vi "SerialTranscieve.vi"(8 "error in (no error)":errorcluster, 9 "TimeOut(ms)":u32=1000, 10 "ByteArrayToSend":u8[](array[numeric])=[126, 0, 0, 2, 0, 3, 250, 126] format="%x", 11 "VISA resource name":refnum<visa-resource-name>="COM7") -> (0 "error out":errorcluster={"status"=TRUE, "code"=-5000, "source"="Serial Transcieve Timout"}, 1 "return count":u32, 2 "ByteArrayRecieved":u8[](array[numeric]), 3 "VISA resource name out":refnum<visa-resource-name>="COM7")   [LabVIEW 2019]
panel:
  out "Numeric":i32
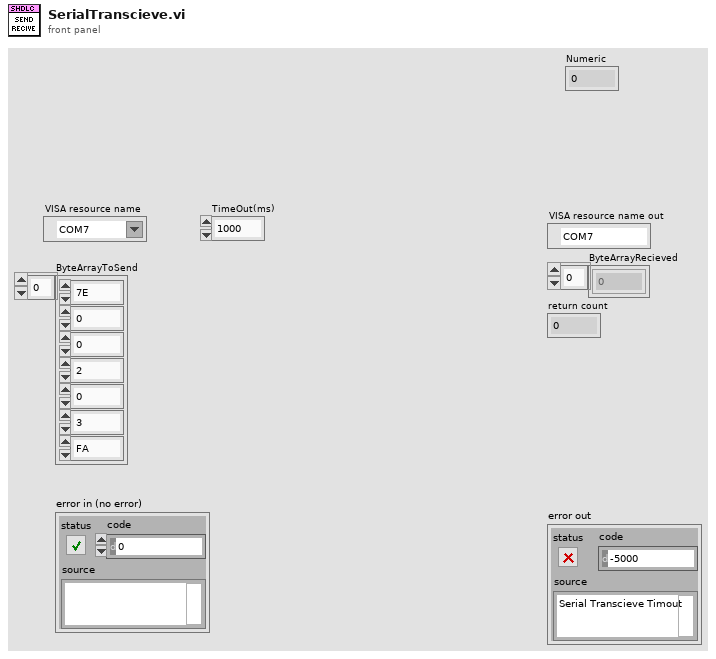
[diagram p1: front panel]
types:
  T1 = enum16{"big-endian, network order", "native, host order", "little-endian"}
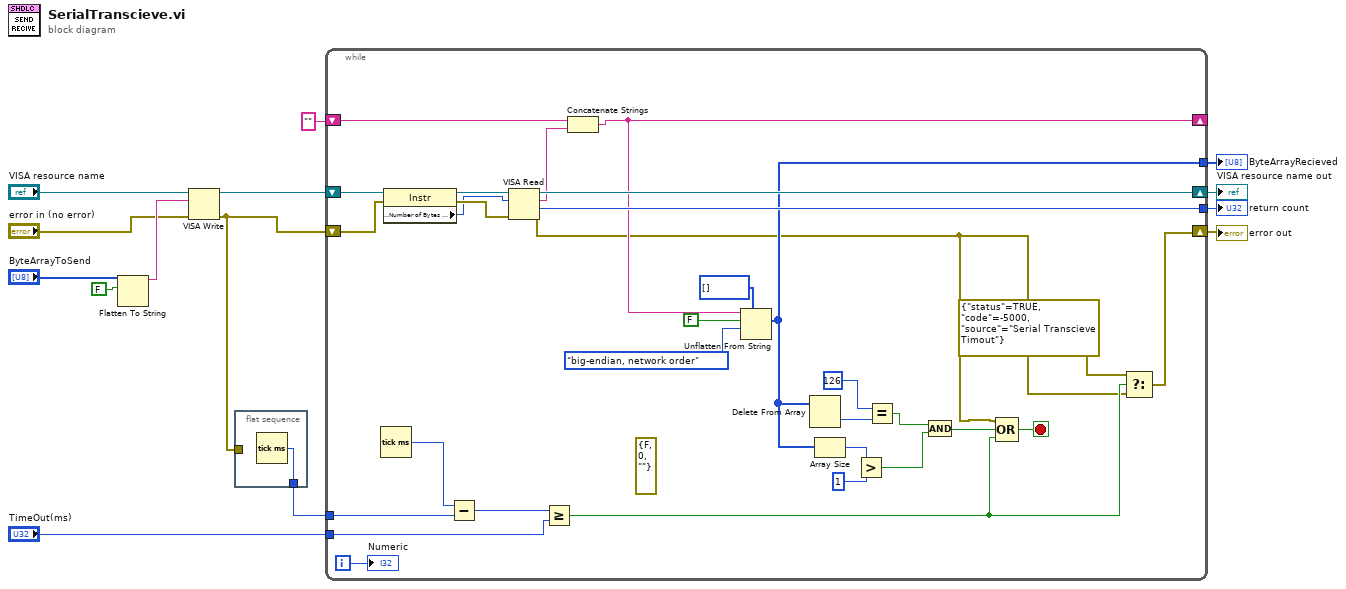
[diagram p0: block diagram]
diagram:
  n1 = Flatten To String(anything="ByteArrayToSend", prepend array or string size? (T)=FALSE) -> (data string=w14:string)  [unwired: 2 in, 2 out]
  n2 = VISA Write(VISA resource name="VISA resource name", write buffer=w14, error in (no error)="error in (no error)") -> (VISA resource name out=w9:refnum<visa-resource-name>, error out=w1:errorcluster)  [unwired: 1 out]
  n3 = flat-sequence {
    tunnel: [w15] -> w2
    tunnel: w1 -> [_]
    frame #0 {
      n4 = Tick Count (ms)() -> (millisecond timer value=w15:u32)
    }
  }
  n5 = while {
    tunnel: [w42] -> w5
    shift-right: [w37] -> w3
    shift-left: w9 -> [w45]
    shift-right: [w17] -> w4
    shift-left: w1 -> [w43]
    shift-right: [w21] -> _
    shift-left: "" -> [w38]
    tunnel: [w28] -> w6
    tunnel: w2 -> [w26]
    tunnel: "TimeOut(ms)" -> [w24]
    i -> [w16]
    stop <- w22 stop-if-true
    (unwired) errorcluster {"status"=FALSE, "code"=0, "source"=""} ("error in (no error)")
    n6 = Tick Count (ms)() -> (millisecond timer value=w27:u32)
    n7 = property class="Instr"(reference=w45, error in=w43) -> (reference out=w46:refnum<visa-resource-name>, error out=w44:errorcluster, "Serial Settings:Number of Bytes at Serial Port"=w29:u32)
    n8 = Subtract(x=w27, y=w26) -> (x-y=w25:u32)
    n9 = VISA Read(VISA resource name=w46, byte count=w29, error in (no error)=w44) -> (VISA resource name out=w37:refnum<visa-resource-name>, read buffer=w30:string, return count=w42:u32, error out=w18:errorcluster)
    n10 = Greater Or Equal?(x=w25, y=w24) -> (x >= y?=w20:bool)
    n11 = Concatenate Strings(w38, w30) -> (w21:string)
    n12 = Unflatten From String(type=u8[] [] ("Array 2"), binary string=w21, data includes array or string size? (T)=FALSE, byte order (0:big-endian, network order)=T1."big-endian, network order") -> (value=w28:u8[])  [unwired: 1 in, 2 out]
    n13 = Delete From Array(array=w28) -> (deleted portion=w36:u8)  [unwired: 2 in, 1 out]
    n14 = Array Size(array=w28) -> (size(s)=w34:i32)
    n15 = Greater?(x=w34, y=1) -> (0:w31:bool)
    n16 = Equal?(x=u8 126 ("Numeric"), y=w36) -> (x = y?=w32:bool)
    n17 = Compound Arithmetic op=AND(w32, w31) -> (w23:bool)
    n18 = Compound Arithmetic op=OR(w18, w23, w20) -> (w22:bool)
    n19 = Select(t=errorcluster {"status"=TRUE, "code"=-5000, "source"="Serial Transcieve Timout"} ("error in (no error)"), s=w20, f=w18) -> (s? t:f=w17:errorcluster)
    "Numeric" <- w16
  }
  "ByteArrayRecieved" <- w6
  "return count" <- w5
  "error out" <- w4
  "VISA resource name out" <- w3
